vi "Main.vi"(8 "error in":errorcluster, 11 "Head Worker in":refnum<class "Head Worker.lvclass">) -> (0 "error out":errorcluster, 3 "Head Worker out":refnum<class "Head Worker.lvclass">)   [LabVIEW 2017, in "Head Worker.lvclass"]
doc: "The <b>Queued Message Handler</b> of the Worker that owns this VI."
uses:
  Head Worker.lvclass
  C:/Program Files (x86)/National Instruments/LabVIEW 2017/vi.lib/addons/_Workers/Library/Classes/Worker/Worker.lvclass
  C:/Users/Peter Scarfe/Documents/LabVIEW Data/New folder (3)/Workers/Base Classes/Worker Base Class/Worker Base Class.lvclass
  Head Worker.lvclass/Head Worker.ctl
  Initialization Data.ctl
  Response Cases.ctl
  subWorker Level 1/subWorker Level 1.lvclass
  Base Classes/Worker Base Class/Worker Base Class.lvclass
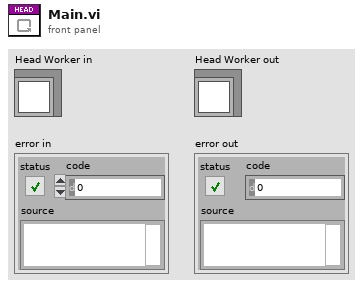
[diagram p1: front panel]
types:
  T1 = typedef "Head Worker.lvclass/Initialization Data.ctl" = cluster{"Response Cases":T2}
  T2 = typedef "Head Worker.lvclass/Response Cases.ctl" = cluster{"Placeholder - Can be deleted":string}
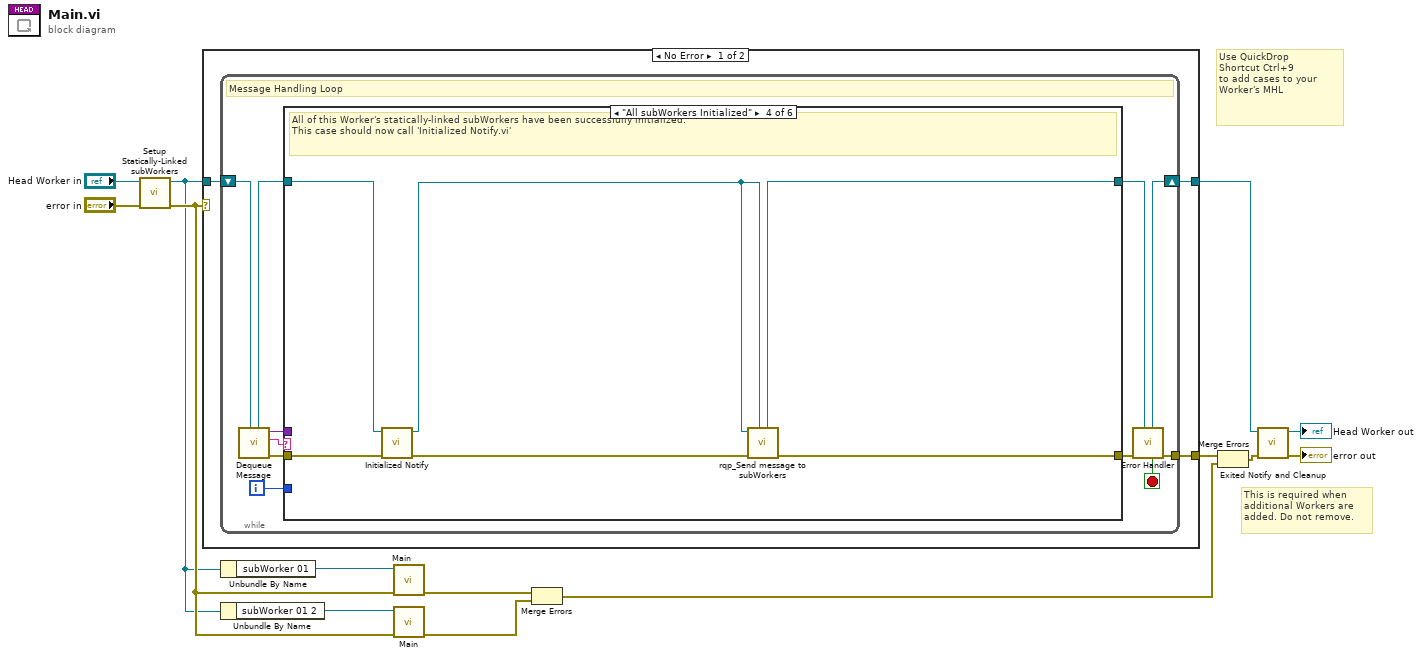
[diagram p0: block diagram]
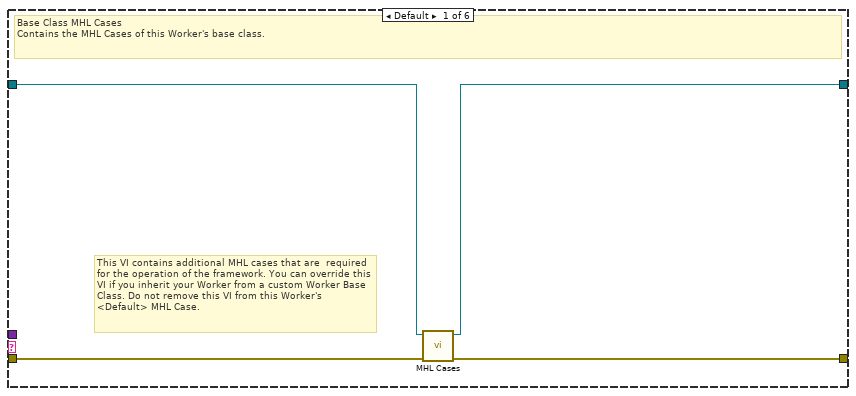
[diagram p2: hidden frame]
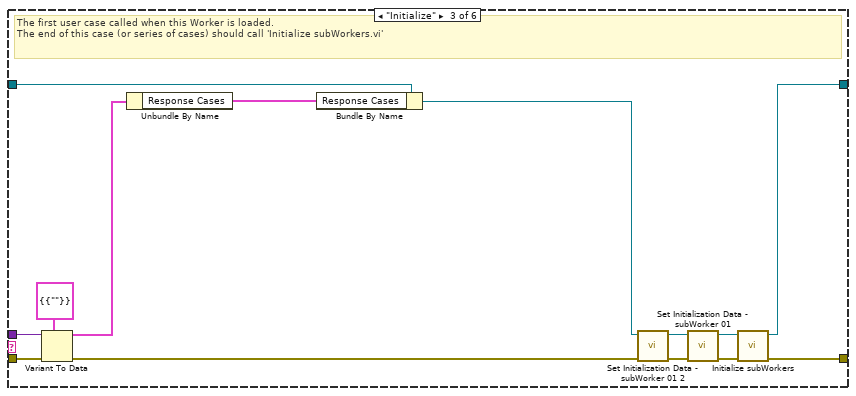
[diagram p4: hidden frame]
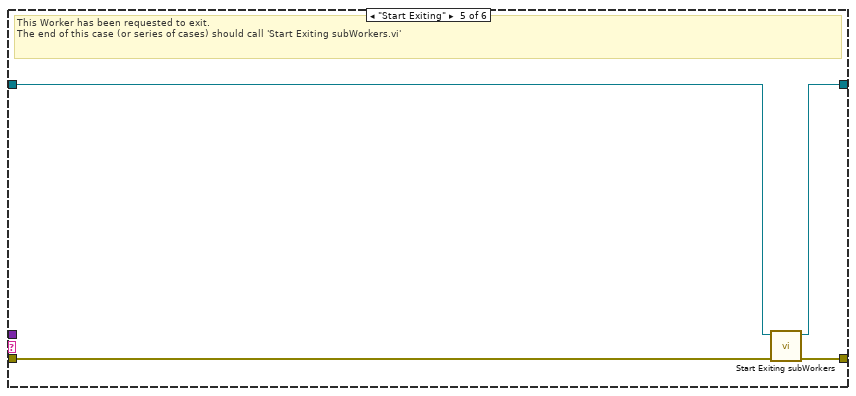
[diagram p5: hidden frame]
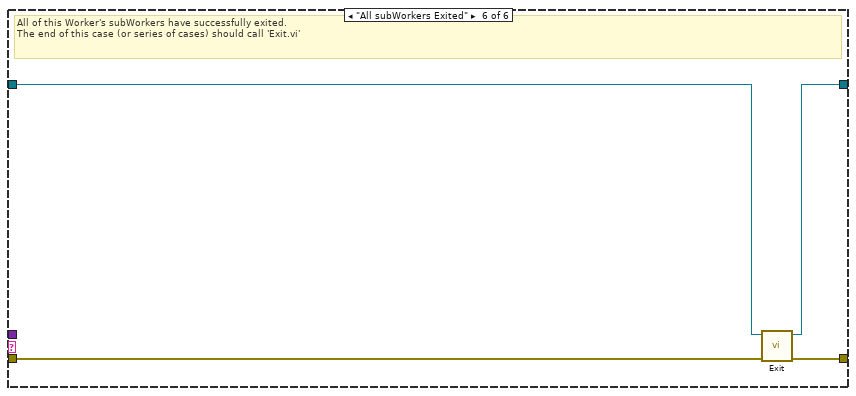
[diagram p6: hidden frame]
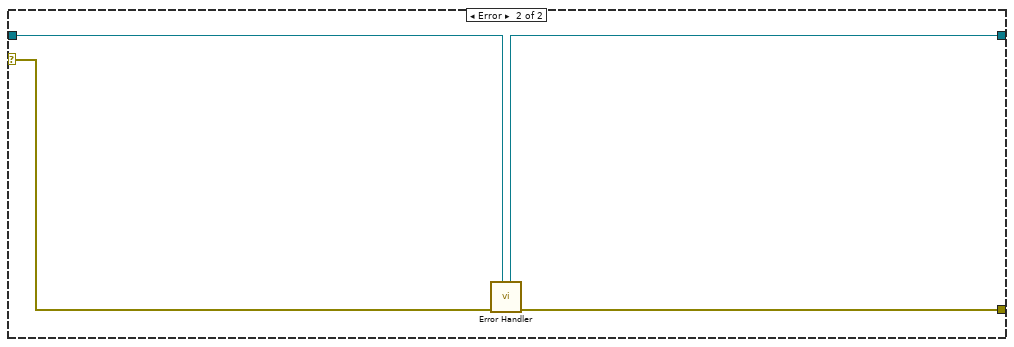
[diagram p7: hidden frame]
diagram:
  # "Use QuickDrop\nShortcut Ctrl+9\nto add cases to your\nWorker's MHL"
  # "This is required when additional Workers are added. Do not remove."
  n1 = call "Setup Statically-Linked subWorkers.vi"("error in"="error in", "Head Worker in"="Head Worker in") -> ("error out"=w8:errorcluster, "Head Worker out"=w6:refnum<class "Head Worker.lvclass">)  [unwired: 8 in]
  n2 = case shown="No Error" w8 {
    tunnel: w6 -> [w15 w64]
    tunnel: [w17 w65] -> w13
    tunnel: [w16 w63] -> w14
    selector: w8 -> [_ w66]
    frame No Error {
      n3 = while {
        shift-right: [w26] -> w16
        shift-left: w15 -> [w28]
        tunnel: [w27] -> w17
        i -> [w18]
        stop <- w19 stop-if-true
        # "Message Handling Loop"
        n4 = call-dynamic "Dequeue Message.vi"("Worker"=w28) -> ("error out"=w25:errorcluster, "Case out"=w20:string, "Data out"=w21:variant, "Worker out"=w23:refnum<class "Head Worker.lvclass">)  [unwired: 6 in, 1 out]
        n5 = case "Worker MHL Case Structure (DO NOT CHANGE LABEL NAME)" shown="\"All subWorkers Initialized\"" w20 {
          tunnel: w25 -> [w32 w33 w46 w54 w55 w62]
          tunnel: [w31 w33 w48 w51 w58 w61] -> w24
          tunnel: w23 -> [w30 w34 w45 w52 w56 w60]
          tunnel: [w29 w34 w47 w50 w57 w59] -> w22
          tunnel: w21 -> [_ _ w43 _ _ _]
          tunnel: w18 -> [_ _ _ _ _ _]
          frame Default {
            # "This VI contains additional MHL cases that are  required for the operation of the framework. You can override this VI if you inherit your Worker from a custom Worker Base Class. Do not remove this VI from this Worker's <Default> MHL Case."
            # "Base Class MHL Cases\nContains the MHL Cases of this Worker's base class."
            n6 = call-dynamic "MHL Cases.vi"("error in"=w32, "Worker Base Class in"=w30) -> ("error out"=w31:errorcluster, "Worker Base Class out"=w29:refnum<class "Head Worker.lvclass">)  [unwired: 8 in]
          }
          frame "------------ FRAMEWORK CASES -----------" {
            # "Start of Workers Framework Cases"
          }
          frame "Initialize" {
            # "The first user case called when this Worker is loaded.\nThe end of this case (or series of cases) should call 'Initialize subWorkers.vi'"
            n7 = Variant To Data(error in=w46, type=T1 {"Response Cases"={"Placeholder - Can be deleted"=""}} ("Cluster"), Variant=w43) -> (data=w42:T1, error out=w44:errorcluster)
            n8 = Unbundle By Name(w42) -> ("Response Cases"=w41:T2)
            n9 = Bundle By Name(cluster=w45, "Response Cases"=w41) -> (w36:refnum<class "Head Worker.lvclass">)
            n10 = call "Set Initialization Data - subWorker 01 2.vi"("error in"=w44, "Head Worker in"=w36) -> ("error out"=w37:errorcluster, "Head Worker out"=w35:refnum<class "Head Worker.lvclass">)  [unwired: 8 in]
            n11 = call "Set Initialization Data - subWorker 01.vi"("error in"=w37, "Head Worker in"=w35) -> ("error out"=w39:errorcluster, "Head Worker out"=w38:refnum<class "Head Worker.lvclass">)  [unwired: 8 in]
            n12 = call-dynamic "Initialize subWorkers.vi"("error in"=w39, "Worker"=w38) -> ("error out"=w48:errorcluster, "dup Worker out"=w47:refnum<class "Head Worker.lvclass">)  [unwired: 8 in]
          }
          frame "All subWorkers Initialized" {
            # "All of this Worker's statically-linked subWorkers have been successfully initialized.\nThis case should now call 'Initialized Notify.vi'"
            n13 = call-dynamic "Initialized Notify.vi"("error in"=w54, "Worker"=w52) -> ("error out"=w53:errorcluster, "dup Worker out"=w49:refnum<class "Head Worker.lvclass">)  [unwired: 8 in]
            n14 = call "rqp_Send message to subWorkers.vi"("Caller in"=w49, "error in"=w53, "Worker Base Class in"=w49) -> ("error out"=w51:errorcluster, "dup Caller out"=w50:refnum<class "Head Worker.lvclass">)  [unwired: 6 in, 1 out]
          }
          frame "Start Exiting" {
            # "This Worker has been requested to exit. \nThe end of this case (or series of cases) should call 'Start Exiting subWorkers.vi'"
            n15 = call-dynamic "Start Exiting subWorkers.vi"("error_in"=w55, "Worker"=w56) -> ("error out"=w58:errorcluster, "dup Worker out"=w57:refnum<class "Head Worker.lvclass">)  [unwired: 8 in]
          }
          frame "All subWorkers Exited" {
            # "All of this Worker's subWorkers have successfully exited. \nThe end of this case (or series of cases) should call 'Exit.vi'"
            n16 = call-dynamic "Exit.vi"("error_in"=w62, "Worker"=w60) -> ("error out"=w61:errorcluster, "dup Worker out"=w59:refnum<class "Head Worker.lvclass">)  [unwired: 8 in]
          }
        }
        n17 = call-dynamic "Error Handler.vi"("Worker"=w22, "error_in"=w24) -> ("error out"=w27:errorcluster, "Stop Loop"=w19:bool, "Worker out"=w26:refnum<class "Head Worker.lvclass">)  [unwired: 7 in]
      }
    }
    frame Error {
      n18 = call-dynamic "Error Handler.vi"("Worker"=w64, "error_in"=w66) -> ("error out"=w65:errorcluster, "Worker out"=w63:refnum<class "Head Worker.lvclass">)  [unwired: 7 in, 1 out]
    }
  }
  n19 = Unbundle By Name(w6) -> ("subWorker 01"=w3:refnum<class "subWorker Level 1.lvclass">)
  n20 = Unbundle By Name(w6) -> ("subWorker 01 2"=w1:refnum<class "subWorker Level 1.lvclass">)
  n21 = call-dynamic "Main.vi"("error in"=w8, "subWorker Level 1 in"=w3) -> ("error out"=w5:errorcluster)  [unwired: 8 in, 1 out]
  n22 = call-dynamic "Main.vi"("error in"=w8, "subWorker Level 1 in"=w1) -> ("error out"=w2:errorcluster)  [unwired: 8 in, 1 out]
  n23 = Merge Errors(w5, w2) -> (w4:errorcluster)
  n24 = Merge Errors(w13, w4) -> (w10:errorcluster)
  n25 = call-dynamic "Exited Notify and Cleanup.vi"("error_in"=w10, "Worker"=w14) -> ("error out"=→"error out":errorcluster, "dup Worker out"=→"Head Worker out":refnum<class "Head Worker.lvclass">)  [unwired: 8 in]
